vi "Graph.vi"(8 "error in (no error)":errorcluster, 11 "Experiment2D in":refnum<class "Experiment2D.lvclass">) -> (0 "error out":errorcluster, 1 "Y":dbl[](array[numeric]), 2 "X":dbl[](array[numeric]), 3 "Experiment2D out":refnum<class "Experiment2D.lvclass">)   [LabVIEW 2014, in "Experiment2D.lvclass"]
uses:
  Experiment2D.lvclass
  Data/Data2D/Data2D.lvclass
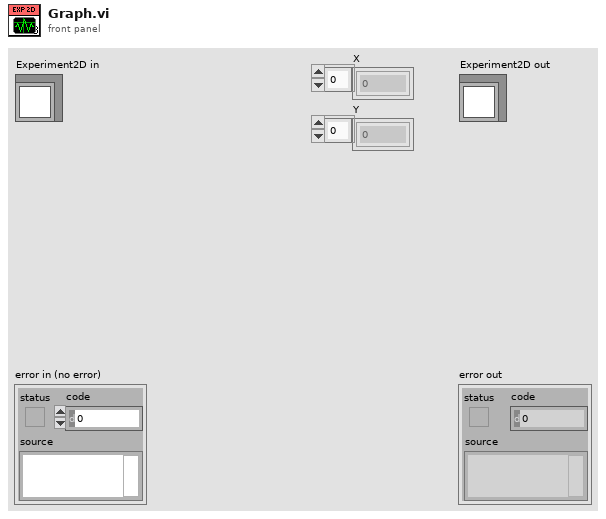
[diagram p1: front panel]
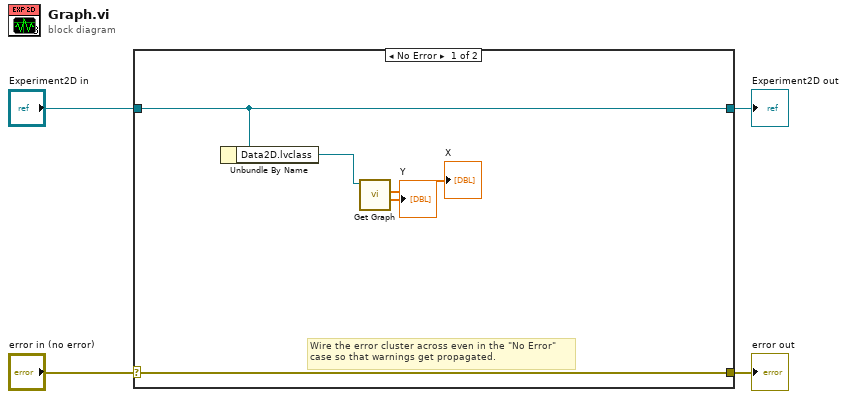
[diagram p0: block diagram]
diagram:
  n1 = case shown="No Error" "error in (no error)" {
    selector: "error in (no error)" -> [w9 w11]
    tunnel: [w9 w11] -> w3
    tunnel: [w8 w10] -> w1
    tunnel: "Experiment2D in" -> [w8 w10]
    frame No Error {
      # "Wire the error cluster across even in the \"No Error\"\ncase so that warnings get propagated."
      n2 = Unbundle By Name(w8) -> ("Data2D.lvclass"=w7:refnum<class "Data2D.lvclass">)
      n3 = call-dynamic "Get Graph.vi"("Data2D in"=w7) -> ("Y"=→"Y":dbl[], "X"=→"X":dbl[])  [unwired: 7 in, 2 out]
    }
    frame Error {
    }
  }
  "error out" <- w3
  "Experiment2D out" <- w1
